vi "closeTestStandStep.vi"(8 "error in":errorcluster, 10 "NewStep":refnum<k7>, 11 "Sequence File Ref":refnum<k7>) -> (0 "error out":errorcluster, 3 "Sequence File Ref(out)":refnum<k7>)   [LabVIEW 2010]
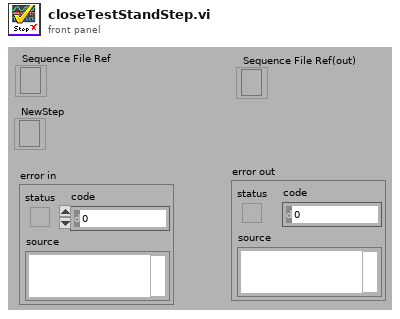
[diagram p1: front panel]
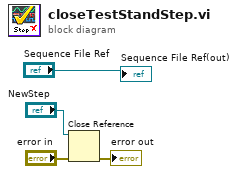
[diagram p0: block diagram]
diagram:
  n1 = Close Reference(reference="NewStep", error in (no error)="error in") -> (error out=→"error out":errorcluster)
  "Sequence File Ref(out)" <- "Sequence File Ref"
